vi "Estimated Time Required.vi"(1 "Lithography Data":T2(array[cluster])) -> (0 "Estimated Time Required":timestamp format="%<%I:%M:%S>T")   [LabVIEW 2019]
doc: "This VI calculates the time required to complete lithography."
uses:
  <userlib>/LevyLab/Relay Box/Typedefs/Resistor--enum.ctl
  <userlib>/LevyLab/Relay Box/Relay-Box.lvclass
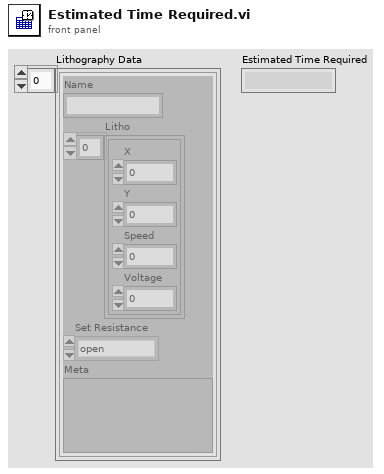
[diagram p1: front panel]
types:
  T1 = typedef "Relay-Box.lvclass/Resistor--enum.ctl" = enum16{"open", "discharge tip", "0 ohms", "100k ohm", "10M ohm", "1G ohm"}
  T2 = cluster{"Name":string, "Litho":cluster{"X":dbl, "Y":dbl, "Speed":dbl, "Voltage":dbl}[], "Set Resistance":T1, "Meta":variant}[]
  T3 = cluster{"X":dbl, "Y":dbl, "Speed":dbl, "Voltage":dbl}[]
  T4 = cluster{"X":dbl, "Y":dbl, "Speed":dbl, "Voltage":dbl}
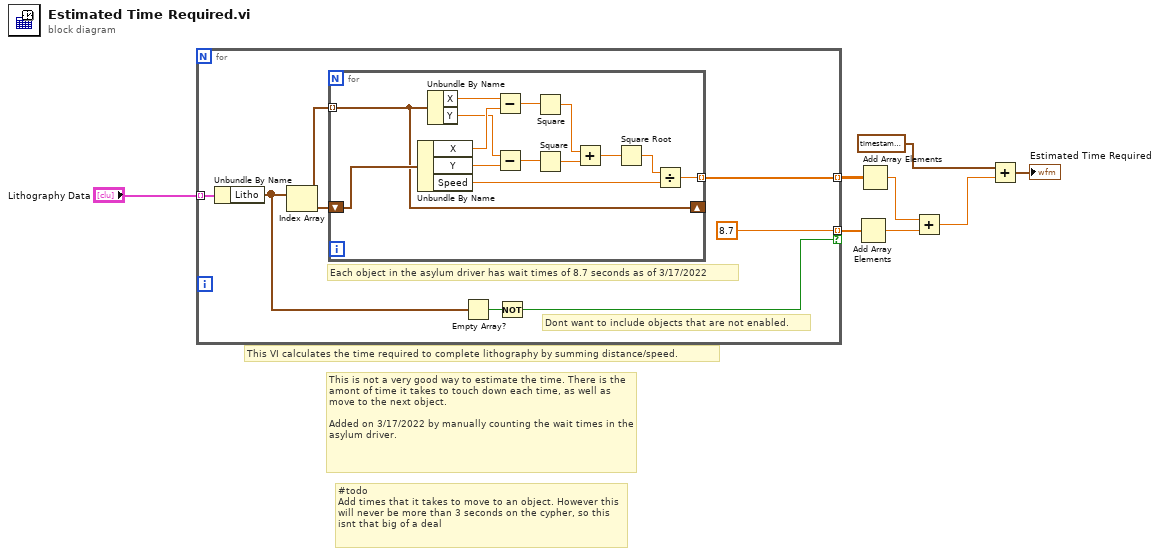
[diagram p0: block diagram]
diagram:
  # "#todo\nAdd times that it takes to move to an object. However this will never be more than 3 seconds on the cypher, so this isnt that big of a deal"
  # "This is not a very good way to estimate the time. There is the amont of time it takes to touch down each time, as well as move to the next object. \n\nAdded on 3/17/2022 by manually counting the wait times in the asylum driver."
  # "This VI calculates the time required to complete lithography by summing distance/speed."
  n1 = for {
    tunnel: "Lithography Data" -> [w15] mode=indexing
    tunnel: [w14] -> w7 mode=indexing
    tunnel: [8.7 ("y")] -> w2 mode=indexing if=w9
    # "Dont want to include objects that are not enabled."
    # "Each object in the asylum driver has wait times of 8.7 seconds as of 3/17/2022"
    n2 = Unbundle By Name(w15) -> ("Litho"=w11:T3)
    n3 = Index Array(array=w11) -> (element=w12:T4)  [unwired: 1 in]
    n4 = for {
      tunnel: w11 -> [w16] mode=indexing
      tunnel: [w25] -> w14 mode=indexing
      shift-right: [w16] -> _
      shift-left: w12 -> [w17]
      n5 = Unbundle By Name(w17) -> ("X"=w23:dbl, "Y"=w20:dbl, "Speed"=w18:dbl)
      n6 = Unbundle By Name(w16) -> ("X"=w24:dbl, "Y"=w21:dbl)
      n7 = Subtract(x=w24, y=w23) -> (x-y=w22:dbl)
      n8 = Subtract(x=w21, y=w20) -> (x-y=w19:dbl)
      n9 = Square(x=w22) -> (x^2=w29:dbl)
      n10 = Square(x=w19) -> (x^2=w28:dbl)
      n11 = Add(x=w29, y=w28) -> (x+y=w27:dbl)
      n12 = Square Root(x=w27) -> (sqrt(x)=w26:dbl)
      n13 = Divide(x=w26, y=w18) -> (x/y=w25:dbl)
    }
    n14 = Empty Array?(array=w11) -> (empty?=w10:bool)
    n15 = Not(x=w10) -> (.not. x?=w9:bool)
  }
  n16 = Add Array Elements(numeric array=w2) -> (sum=w1:dbl)
  n17 = Add Array Elements(numeric array=w7) -> (sum=w4:dbl)
  n18 = Add(x=w4, y=w1) -> (x+y=w3:dbl)
  n19 = Add(x=timestamp(-68400 s since 1904-01-01), y=w3) -> (x+y=→"Estimated Time Required":timestamp)
